vi "SDO_DRIVE_MODULE_OPEN.vi"(3 "Module Index":i32, 4 "RadiansPerCount":dbl=1.0, 5 "Drive PWM Channel":T2, 6 "DistancePerCount":dbl=1.0, 7 "Swerve PWM Channel":T2, 8 "Swerve B Channel":T1, 9 "Swerver A Channel":T1, 10 "Drive B Channel":T1, 11 "Drive A channel":T1) -> ()   [LabVIEW 2019]
uses:
  <vilib>/Rock Robotics/WPI/MotorControl/WPI_MotorControlOpen SPARK.vi
  <vilib>/Rock Robotics/WPI/Counter/WPI_CounterDigitalInputToDigitalSource.vi
  <vilib>/Rock Robotics/WPI/SafetyOutput/WPI_SafetyOutputConfigMenu.ctl
  <vilib>/Rock Robotics/WPI/Encoder/WPI_EncoderType.ctl
  <vilib>/Rock Robotics/SystemInterfaces/DIO/FPGA_DIOChannel.ctl
  <vilib>/Rock Robotics/SystemInterfaces/DIO/FPGA_DIOPWMChannel.ctl
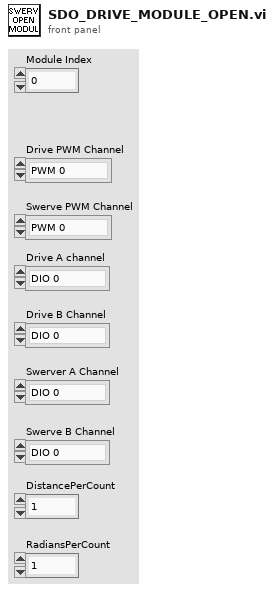
[diagram p1: front panel]
types:
  T1 = typedef "FPGA_DIOChannel.ctl" = enum8{"DIO 0", "DIO 1", "DIO 2", "DIO 3", "DIO 4", "DIO 5", "DIO 6", "DIO 7", "DIO 8", "DIO 9", "DIO MXP 0", "DIO MXP 1", "DIO MXP 2", "DIO MXP 3", "DIO MXP 4", "DIO MXP 5", "DIO MXP 6", "DIO MXP 7", "DIO MXP 8", "DIO MXP 9", "DIO MXP 10", "DIO MXP 11", "DIO MXP 12", "DIO MXP 13", "DIO MXP 14", "DIO MXP 15", "SPI Port CS1", "SPI Port CS2", "SPI Port CS3", "SPI Port MISO", "SPI Port MOSI", "Invalid"}
  T2 = typedef "FPGA_DIOPWMChannel.ctl" = enum8{"PWM 0", "PWM 1", "PWM 2", "PWM 3", "PWM 4", "PWM 5", "PWM 6", "PWM 7", "PWM 8", "PWM 9", "PWM MXP 0", "PWM MXP 1", "PWM MXP 2", "PWM MXP 3", "PWM MXP 4", "PWM MXP 5", "PWM MXP 6", "PWM MXP 7", "PWM MXP 8", "PWM MXP 9", "Invalid"}
  T3 = typedef "WPI_EncoderType.ctl" = enum16{"1x", "2x", "4x"}
  T4 = typedef "WPI_SafetyOutputConfigMenu.ctl" = enum16{"Enable", "Disable"}
  T5 = typedef "WPI_MotorControlDeviceRef.ctl" = cluster{"DeviceStatus":errorcluster, "Type":T6, "PWM":cluster{"PWM Channel":T2, "DeadBand":T7}, "CAN":cluster{"Device Number":u8, "SetOutput VI Ref":variant, "GetOutput VI Ref":variant, "Enable VI Ref":variant, "Disable VI Ref":variant, "Data":variant}, "Invert":bool, "DIO PWM":cluster{"PWM \"Enable\" Channel":T2, "DIOChannel":T1, "PWM Rate":dbl}}
  T6 = typedef "WPI_MotorControlType.ctl" = enum16{"PWM", "CAN", "DIO PWM"}
  T7 = typedef "WPI_PWMDeadband.ctl" = cluster{"Name":string, "maxPositivePwm":i32, "minPositivePwm":i32, "centerPwm":i32, "maxNegativePwm":i32, "minNegativePwm":i32, "angularRange":u16}
  T8 = typedef "WPI_DigitalInputDevRef.ctl" = cluster{"DevStatus":errorcluster, "DIO Channel":T1}
  T9 = typedef "FPGA_CounterEncoderSourceConvertionLVSourceType.ctl" = cluster{"DevStatus":errorcluster, "AnalogTriggerMode?":bool, "DigitalMode":cluster{"DIO Channel":T10}, "AnalogTriggerMode":cluster{"AnalogTriggerIndex":T11, "OutputType":T12}}
  T10 = typedef "FPGA_DIODigitalSourceChannel.ctl" = enum8{"DIO 0", "DIO 1", "DIO 2", "DIO 3", "DIO 4", "DIO 5", "DIO 6", "DIO 7", "DIO 8", "DIO 9", "DIO MXP 0", "DIO MXP 1", "DIO MXP 2", "DIO MXP 3", "DIO MXP 4", "DIO MXP 5", "DIO MXP 6", "DIO MXP 7", "DIO MXP 8", "DIO MXP 9", "DIO MXP 10", "DIO MXP 11", "DIO MXP 12", "DIO MXP 13", "DIO MXP 14", "DIO MXP 15", "SPI Port CS1", "SPI Port CS2", "SPI Port CS3", "SPI Port MISO", "SPI Port MOSI", "Disabled"}
  T11 = typedef "FPGA_AnalogTriggerIndex.ctl" = enum8{"Trig 0", "Trig 1", "Trig 2", "Trig 3", "Trig 4", "Trig 5", "Trig 6", "Trig 7", "Invalid"}
  T12 = typedef "FPGA_AnalogTriggerOutType.ctl" = enum16{"InWindow", "TriggerState", "Rising", "Falling"}
  T13 = typedef "WPI_EncoderDevRef.ctl" = cluster{"DevStatus":errorcluster, "EncoderIndex":T14, "CounterIndex":T15, "DistancePerCount":dbl, "Decoding Type":T3}
  T14 = typedef "FPGA_EncoderIdx.ctl" = enum8{"Enc 0", "Enc 1", "Enc 2", "Enc 3", "Enc 4", "Enc 5", "Enc 6", "Enc 7", "Invalid"}
  T15 = typedef "FPGA_CounterCtrSystemIndex.ctl" = enum8{"Ctr 0", "Ctr 1", "Ctr 2", "Ctr 3", "Ctr 4", "Ctr 5", "Ctr 6", "Ctr 7", "Invalid"}
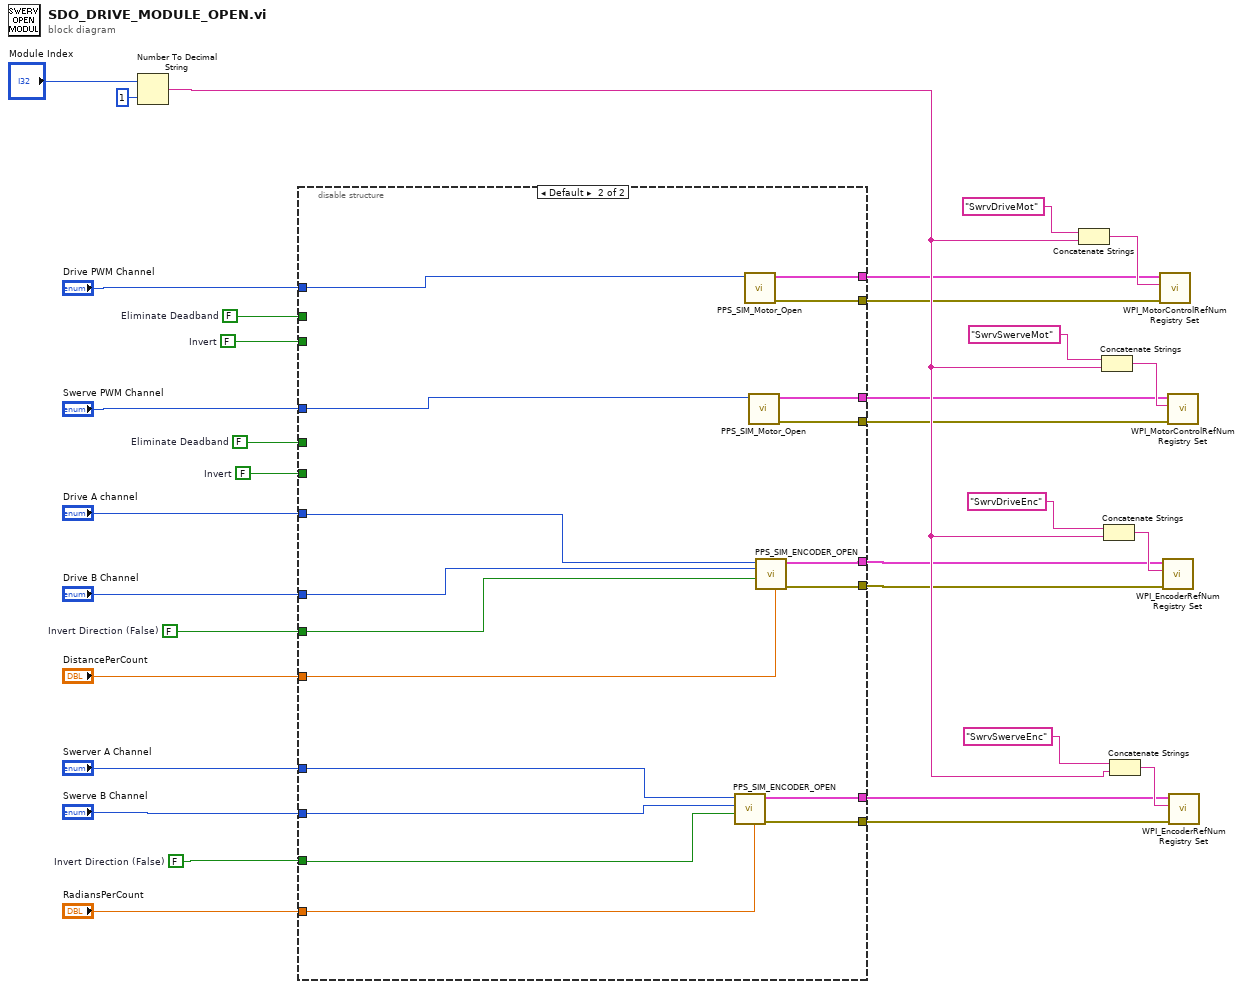
[diagram p0: block diagram]
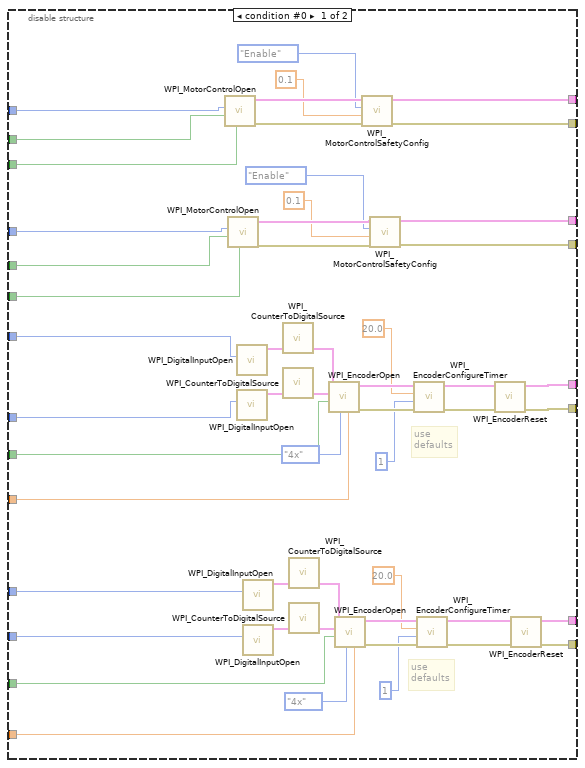
[diagram p2: hidden frame]
diagram:
  w2 = FALSE  # Eliminate Deadband
  w1 = FALSE  # Invert
  w4 = FALSE  # Invert
  w3 = FALSE  # Eliminate Deadband
  w5 = FALSE  # Invert Direction (False)
  w6 = FALSE  # Invert Direction (False)
  n1 = Number To Decimal String(number="Module Index", width (-)=i16 1) -> (decimal integer string=w15:string)
  n2 = disable-structure shown="Default" {
    disable-tunnel: "Swerve B Channel" -> [w67 w95]
    disable-tunnel: "Swerver A Channel" -> [w66 w94]
    disable-tunnel: "RadiansPerCount" -> [w65 w97]
    disable-tunnel: "Drive B Channel" -> [w57 w100]
    disable-tunnel: "Drive A channel" -> [w56 w101]
    disable-tunnel: "DistancePerCount" -> [w55 w98]
    disable-tunnel: "Swerve PWM Channel" -> [w53 w90]
    disable-tunnel: "Drive PWM Channel" -> [w52 w91]
    disable-tunnel: [w49 w86] -> w14
    disable-tunnel: [w48 w87] -> w13
    disable-tunnel: [w47 w88] -> w12
    disable-tunnel: [w46 w89] -> w11
    disable-tunnel: [w43 w102] -> w10
    disable-tunnel: [w42 w103] -> w9
    disable-tunnel: [w41 w92] -> w8
    disable-tunnel: [w40 w93] -> w7
    disable-tunnel: w6 -> [w39 w96]
    disable-tunnel: w5 -> [w38 w99]
    disable-tunnel: w4 -> [w37 _]
    disable-tunnel: w3 -> [w36 _]
    disable-tunnel: w2 -> [w35 _]
    disable-tunnel: w1 -> [w34 _]
    frame condition #0 {
      # "use\ndefaults"
      # "use\ndefaults"
      n3 = call-poly <vilib>:"WPI_MotorControlOpen.vi"("Invert"=w37, "Eliminate Deadband"=w36, "PWM Channel"=w52) -> ("error out"=w80:errorcluster, "MotorControlDeviceRef"=w81:T5)  [unwired: 7 in]
      n4 = call-poly <vilib>:"WPI_MotorControlOpen.vi"("Invert"=w34, "Eliminate Deadband"=w35, "PWM Channel"=w53) -> ("error out"=w78:errorcluster, "MotorControlDeviceRef"=w79:T5)  [unwired: 7 in]
      n5 = call <vilib>:"WPI_DigitalInputOpen.vi"("DIO Channel"=w56) -> ("DigitalInputDevRef"=w83:T8)  [unwired: 1 in, 9 out]
      n6 = call <vilib>:"WPI_DigitalInputOpen.vi"("DIO Channel"=w57) -> ("DigitalInputDevRef"=w84:T8)  [unwired: 1 in, 9 out]
      n7 = call <vilib>:"WPI_DigitalInputOpen.vi"("DIO Channel"=w66) -> ("DigitalInputDevRef"=w73:T8)  [unwired: 1 in, 9 out]
      n8 = call <vilib>:"WPI_DigitalInputOpen.vi"("DIO Channel"=w67) -> ("DigitalInputDevRef"=w74:T8)  [unwired: 1 in, 9 out]
      n9 = call-poly <vilib>:"WPI_CounterToDigitalSource.vi"("DigitalInputDevRef"=w83) -> ("Digital Source"=w82:T9)  [unwired: 6 out]
      n10 = call-poly <vilib>:"WPI_CounterToDigitalSource.vi"("DigitalInputDevRef"=w84) -> ("Digital Source"=w85:T9)  [unwired: 6 out]
      n11 = call-poly <vilib>:"WPI_CounterToDigitalSource.vi"("DigitalInputDevRef"=w73) -> ("Digital Source"=w72:T9)  [unwired: 6 out]
      n12 = call-poly <vilib>:"WPI_CounterToDigitalSource.vi"("DigitalInputDevRef"=w74) -> ("Digital Source"=w75:T9)  [unwired: 6 out]
      n13 = call <vilib>:"WPI_EncoderOpen.vi"("DistancePerCount"=w55, "Decoding Type"=WPI_EncoderType."4x", "Invert Direction (False)"=w38, "BSource"=w85, "ASource"=w82) -> ("error out"=w76:errorcluster, "EncoderDevRef"=w77:T13)  [unwired: 3 in, 2 out]
      n14 = call <vilib>:"WPI_EncoderOpen.vi"("DistancePerCount"=w65, "Decoding Type"=WPI_EncoderType."4x", "Invert Direction (False)"=w39, "BSource"=w75, "ASource"=w72) -> ("error out"=w70:errorcluster, "EncoderDevRef"=w71:T13)  [unwired: 3 in, 2 out]
      n15 = call <vilib>:"WPI_MotorControlSafetyConfig.vi"("error in (no error)"=w80, "timeout (s)"=0.1, "mode"=WPI_SafetyOutputConfigMenu."Enable", "MotorControlDevRef"=w81) -> ("error out"=w47:errorcluster, "MotorControlDevRef"=w46:T5)  [unwired: 6 in]
      n16 = call <vilib>:"WPI_MotorControlSafetyConfig.vi"("error in (no error)"=w78, "timeout (s)"=0.1, "mode"=WPI_SafetyOutputConfigMenu."Enable", "MotorControlDevRef"=w79) -> ("error out"=w49:errorcluster, "MotorControlDevRef"=w48:T5)  [unwired: 6 in]
      n17 = call <vilib>:"WPI_EncoderConfigureTimer.vi"("error in (no error)"=w76, "Number Samples to Average"=u8 1, "Minimum Rate"=20.0, "EncoderDevRef"=w77) -> ("error out"=w45:errorcluster, "EncoderDevRef"=w44:T13)  [unwired: 6 in]
      n18 = call <vilib>:"WPI_EncoderConfigureTimer.vi"("error in (no error)"=w70, "Number Samples to Average"=u8 1, "Minimum Rate"=20.0, "EncoderDevRef"=w71) -> ("error out"=w51:errorcluster, "EncoderDevRef"=w50:T13)  [unwired: 6 in]
      n19 = call <vilib>:"WPI_EncoderReset.vi"("error in (no error)"=w45, "EncoderDevRef"=w44) -> ("error out"=w43:errorcluster, "EncoderDevRef"=w42:T13)  [unwired: 8 in]
      n20 = call <vilib>:"WPI_EncoderReset.vi"("error in (no error)"=w51, "EncoderDevRef"=w50) -> ("error out"=w41:errorcluster, "EncoderDevRef"=w40:T13)  [unwired: 8 in]
    }
    frame condition #1 (active) {
      n21 = call "PPS_SIM_ENCODER_OPEN.vi"("DistancePerCount"=w97, "Invert"=w96, "DIO Channel B"=w95, "DIO Channel  A"=w94) -> ("error out"=w92:errorcluster, "SwerveDriveEnc"=w93:T13)  [unwired: 6 in]
      n22 = call "PPS_SIM_Motor_Open.vi"("PWM Channel"=w91) -> ("error out"=w88:errorcluster, "Motor Device Reference"=w89:T5)  [unwired: 9 in]
      n23 = call "PPS_SIM_Motor_Open.vi"("PWM Channel"=w90) -> ("error out"=w86:errorcluster, "Motor Device Reference"=w87:T5)  [unwired: 9 in]
      n24 = call "PPS_SIM_ENCODER_OPEN.vi"("DistancePerCount"=w98, "Invert"=w99, "DIO Channel B"=w100, "DIO Channel  A"=w101) -> ("error out"=w102:errorcluster, "SwerveDriveEnc"=w103:T13)  [unwired: 6 in]
    }
  }
  n25 = Concatenate Strings("SwrvDriveMot" ("refnum name"), w15) -> (w16:string)
  n26 = Concatenate Strings("SwrvSwerveMot" ("refnum name"), w15) -> (w17:string)
  n27 = Concatenate Strings("SwrvDriveEnc" ("refnum name"), w15) -> (w18:string)
  n28 = Concatenate Strings("SwrvSwerveEnc" ("refnum name"), w15) -> (w19:string)
  n29 = call <vilib>:"WPI_MotorControlRefNum Registry Set.vi"("error in (no error)"=w12, "refnum name"=w16, "MotorControlDevRef"=w11) -> ()  [unwired: 7 in, 2 out]
  n30 = call <vilib>:"WPI_EncoderRefNum Registry Set.vi"("error in (no error)"=w10, "refnum name"=w18, "EncoderDevRef"=w9) -> ()  [unwired: 7 in, 2 out]
  n31 = call <vilib>:"WPI_MotorControlRefNum Registry Set.vi"("error in (no error)"=w14, "refnum name"=w17, "MotorControlDevRef"=w13) -> ()  [unwired: 7 in, 2 out]
  n32 = call <vilib>:"WPI_EncoderRefNum Registry Set.vi"("error in (no error)"=w8, "refnum name"=w19, "EncoderDevRef"=w7) -> ()  [unwired: 7 in, 2 out]
